vi "P1Y2.vi"() -> ()   [LabVIEW 2020]
panel:
  out "x/y":dbl
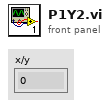
[diagram p1: front panel]
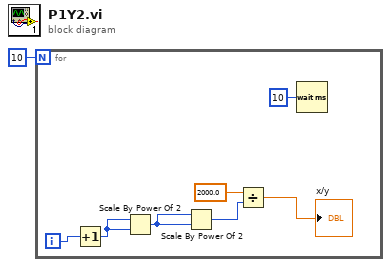
[diagram p0: block diagram]
diagram:
  n1 = for {
    N: 10 -> [_]
    i -> [w8]
    n2 = Increment(x=w8) -> (x+1=w7:i32)
    n3 = Scale By Power Of 2(n=w7, x=w7) -> (x*2^n=w6:i32)
    n4 = Scale By Power Of 2(n=w6, x=w6) -> (x*2^n=w4:i32)
    n5 = Divide(x=2000.0, y=w4) -> (x/y=→"x/y":dbl)
    n6 = Wait (ms)(milliseconds to wait=u32 10) -> ()  [unwired: 1 out]
  }
